vi "Feed Module (Main).vi"(7 "Name of Parent Panel":string="Main.vi", 9 "New Center Coords":T1={"Horizontal"=470, "Vertical"=200}, 10 "Config":variant, 11 "Main UI Message Queue":refnum<queue>) -> ()   [LabVIEW 2018, in "Feed Module.lvlib"]
doc: "This Continuous Measurement sample project is based on the Queued Message Handler template.\n\nThe Event Handling Loop generates messages based on user interface actions.\n\nThe Message Handling Loop processes messages generated by the Event Handling Loop, or by other messages. There are also Acquisition and Logging message handling loop subVIs, and a chart updating loop."
uses:
  Feed Module.lvlib
  support/Message Queue/Message Cluster.ctl
  <vilib>/Utility/miscctls.llb/LVPoint32TypeDef.ctl
  controls/UI Data.ctl
  controls/UI State.ctl
  Controls/Feed Module Config Cluster.ctl
  Controls/Feed Module Settings Cluster.ctl
  Ismatec ISM 831C/Controls/Ismatech Settings Cluster.ctl
  Masterflex 7550-30/Controls/Settings Cluster.ctl
  Mettler Toledo/Controls/Settings Cluster.ctl
  Bronkhorst M13 Flow Meter/Settings Cluster.ctl
  Measure Instrument/PID 2 Parameters Cluster.ctl
  Measure Instrument/PID Input Enum.ctl
  Measure Instrument/PID 2 Output Enum.ctl
  Tacmina QI/Tacmina QI DAQ Setting.ctl
  KNF Pump/Settings Cluster plus SIMDOS.ctl
  ASIA Pump/Pump Settings.ctl
  VICI M50 Party Mode/Settings Cluster.ctl
  FLOM Pump/Settings Cluster.ctl
  SSI PR Class/SSI PR Settings Cluster.ctl
  Controls/Feed Module State Cluster.ctl
  Controls/Feed Module Shared Variable Cluster.ctl
  Controls/Feed Module Display.ctl
  Sequencing/Squence Update Cluster.ctl
  support/Message Queue/Enqueue Message (Single).vi
  <vilib>/Utility/error.llb/Error Cluster From Error Code.vi
  <vilib>/ErrorRing/Error Ring.xnode
  support/User Event - Stop/User Event - Stop.lvlib
  support/Support Library.lvlib
  support/Message Queue/Message Queue.lvlib
  Measure Instrument/Feed Module Engine.lvlib
  Bronkhorst M13 Flow Meter/Bronkhorst M13 Flow Meter.lvlib
  Mettler Toledo/Mettler Toledo.lvlib
  Masterflex 7550-30/Masterflex 7550-30.lvlib
  Ismatec ISM 831C/Ismatec ISM 831C.lvlib
  Operation Window.vi
  Tacmina QI/Tacmina QI.lvlib
  KNF Pump/KNF SIMDOS.lvlib
  ASIA Pump.lvlib
  Sequencing/Sequencing Library.lvlib
  VICI M50 Party Mode/VICI M6 M50 Party Mode.lvlib
  FLOM Pump/FLOM Pump.lvlib
  support/Command Log VIs/Command Logging.lvlib
  SSI PR Class/SSI PR Pump.lvlib
panel:
  out "Pump Flow":dbl
  out "PSIG":dbl format="%#_4g"
  in  "Operation Window":bool
  out "Flow":dbl caption="g/min" format="%.2f"
  out "Ring":u16(ring)=2
  out "Log File path":path
  out "Status":string
  in  "Exit":bool
  out "kg/m^3":dbl format="%#1_4g"
  out "g":dbl format="%#_4g"
  out "C":dbl format="%#_4g"
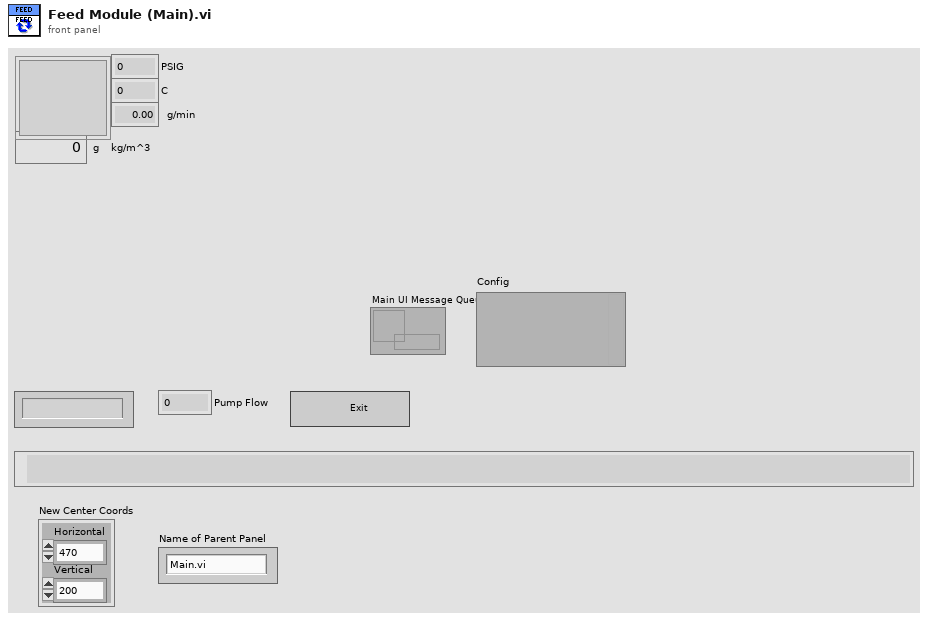
[diagram p1: front panel]
types:
  T1 = typedef "LVPoint32TypeDef.ctl" = cluster{"Horizontal":i32, "Vertical":i32}
  T2 = typedef "Feed Module.lvlib/Feed Module State Cluster.ctl" = cluster{"Shared Variables":T3, "Feed Module Config":T4}
  T3 = typedef "Feed Module.lvlib/Feed Module Shared Variable Cluster.ctl" = cluster{"PID 1 Process Variable":string, "PID 1 Output":string, "PID 1 Setpoint":string, "PID 1 Setpoint SV refnum":refnum<k21>, "PID 1 Process Variable SV refnum":refnum<k21>, "PID 1 Output SV refnum":refnum<k21>}
  T4 = typedef "Feed Module.lvlib/Feed Module Config Cluster.ctl" = cluster{"GUID":string, "Drop Coords":T1, "Process Name":string, "Settings":T5, "Settings Load Count":i32, "OP Load Count":i32}
  T5 = typedef "Feed Module.lvlib/Feed Module Settings Cluster.ctl" = cluster{"Cycle Period":dbl, "Ismatech":T6, "Masterflex":T7, "Mettler":T8, "Bronkhorst M13 Flow Meter":T9, "PID 2 Parameters":T10, "Manual Entry":dbl, "Auto?":bool, "output range":cluster{"output high":dbl, "output low":dbl}, "Bronkhorst M14":T8, "Tacmina Settings":T13, "KNF SIMDOS Settings":T14, "ASIA Pump C":T15, "VICI Settings":T16, "FLOM Settings":T17, "SSI PR Settings":T18}
  T6 = typedef "Ismatec ISM 831C.lvlib/Ismatech Settings Cluster.ctl" = cluster{"VISA resource name":refnum<visa-resource-name>, "Simulated?":bool, "Pump Number":dbl, "Reverse?":bool}
  T7 = typedef "Masterflex 7550-30.lvlib/Settings Cluster.ctl" = cluster{"VISA resource name":refnum<visa-resource-name>, "Simulated?":bool, "Pump Number":dbl, "Reverse?":bool}
  T8 = typedef "Mettler Toledo.lvlib/Settings Cluster.ctl" = cluster{"VISA resource name":refnum<visa-resource-name>, "Simulated?":bool}
  T9 = typedef "Bronkhorst M13 Flow Meter.lvlib/Settings Cluster.ctl" = cluster{"VISA resource name":refnum<visa-resource-name>, "Simulated?":bool}
  T10 = typedef "PID 2 Parameters Cluster.ctl" = cluster{"Input Device":T11, "Output Device":T12, "Setpoint":dbl, "PID gains":cluster{"proportional gain (Kc)":dbl, "integral time (Ti, min)":dbl, "derivative time (Td, min)":dbl}}
  T11 = typedef "PID Input Enum.ctl" = enum16{"Default", "Bronkhorst M13", "Bronkhorst M14", "Scale Rate of Change"}
  T12 = typedef "PID 2 Output Enum.ctl" = enum16{"Default", "Ismatec ISM 831C", "Masterflex 7550-30", "VICI", "Tacmina QI", "KNF SIMDOS", "ASIA Type C", "FLOM UI-22-11", "SSI PR"}
  T13 = typedef "Tacmina QI.lvlib/Tacmina QI DAQ Setting.ctl" = cluster{"Analog DAQ Task":refnum<k21>, "Digital DAQ Task":refnum<k21>}
  T14 = typedef "KNF SIMDOS.lvlib/Settings Cluster plus SIMDOS.ctl" = cluster{"VISA resource name":refnum<visa-resource-name>, "Simulated?":bool}
  T15 = typedef "ASIA Pump.lvlib/Pump Settings.ctl" = cluster{"ASIA Pump #":i32, "channel":i32, "Simulated":bool}
  T16 = typedef "VICI M6 M50 Party Mode.lvlib/Settings Cluster.ctl" = cluster{"VISA resource name":refnum<visa-resource-name>, "Simulated?":bool, "Pump Letter":string, "Reverse?":bool}
  T17 = typedef "FLOM Pump.lvlib/Settings Cluster.ctl" = cluster{"VISA resource name":refnum<visa-resource-name>, "Simulated?":bool, "Pump Number":dbl}
  T18 = typedef "SSI PR Pump.lvlib/SSI PR Settings Cluster.ctl" = cluster{"VISA resource name":refnum<visa-resource-name>, "Simulated?":bool}
  T19 = typedef "UI State.ctl" = enum16{"Idle", "Acquiring and Logging", "Waiting for Exit", "Waiting for Exit (Acq Stopped)", "Waiting for Exit (Log Stopped)", "Waiting for Stop", "Waiting for Stop (Acq Stopped)", "Waiting for Stop (Log Stopped)"}
  T20 = typedef "UI Data.ctl" = cluster{"Start Ref":refnum<vi>, "Trigger Ref":refnum<vi>, "Stop Ref":refnum<vi>, "Settings Ref":refnum<vi>, "Status Ref":refnum<vi>, "Exit Ref":refnum<vi>, "Data Ref":refnum<vi>}
  T21 = typedef "Feed Module.lvlib/Feed Message Queues.ctl" = cluster{"UI":refnum<queue>, "Engine":refnum<queue>, "FM Display":refnum<queue>, "OP Display":refnum<queue>}
  T22 = typedef "Feed Module.lvlib/Feed Module Display.ctl" = cluster{"Flow":dbl, "Density":dbl, "FL Temp":dbl, "Scale Value":dbl, "Pump On?":enum16{"Off", "On", "Not Initialized"}, "Cycle Period":dbl, "Input Device":T11, "Output":T12, "Pump's Pressure":dbl, "Pump's Flow ":dbl}
  T23 = cluster{"Shift":bool, "Ctrl":bool, "Alt":bool, "Cmd":bool, "Opt":bool}
  T24 = typedef "Sequencing Library.lvlib/Squence Update Cluster.ctl" = cluster{"Auto?":bool, "Manual Entry":dbl, "Setpoint":dbl}
  T25 = enum8{"Enabled", "Disabled", "Disabled and Grayed Out"}
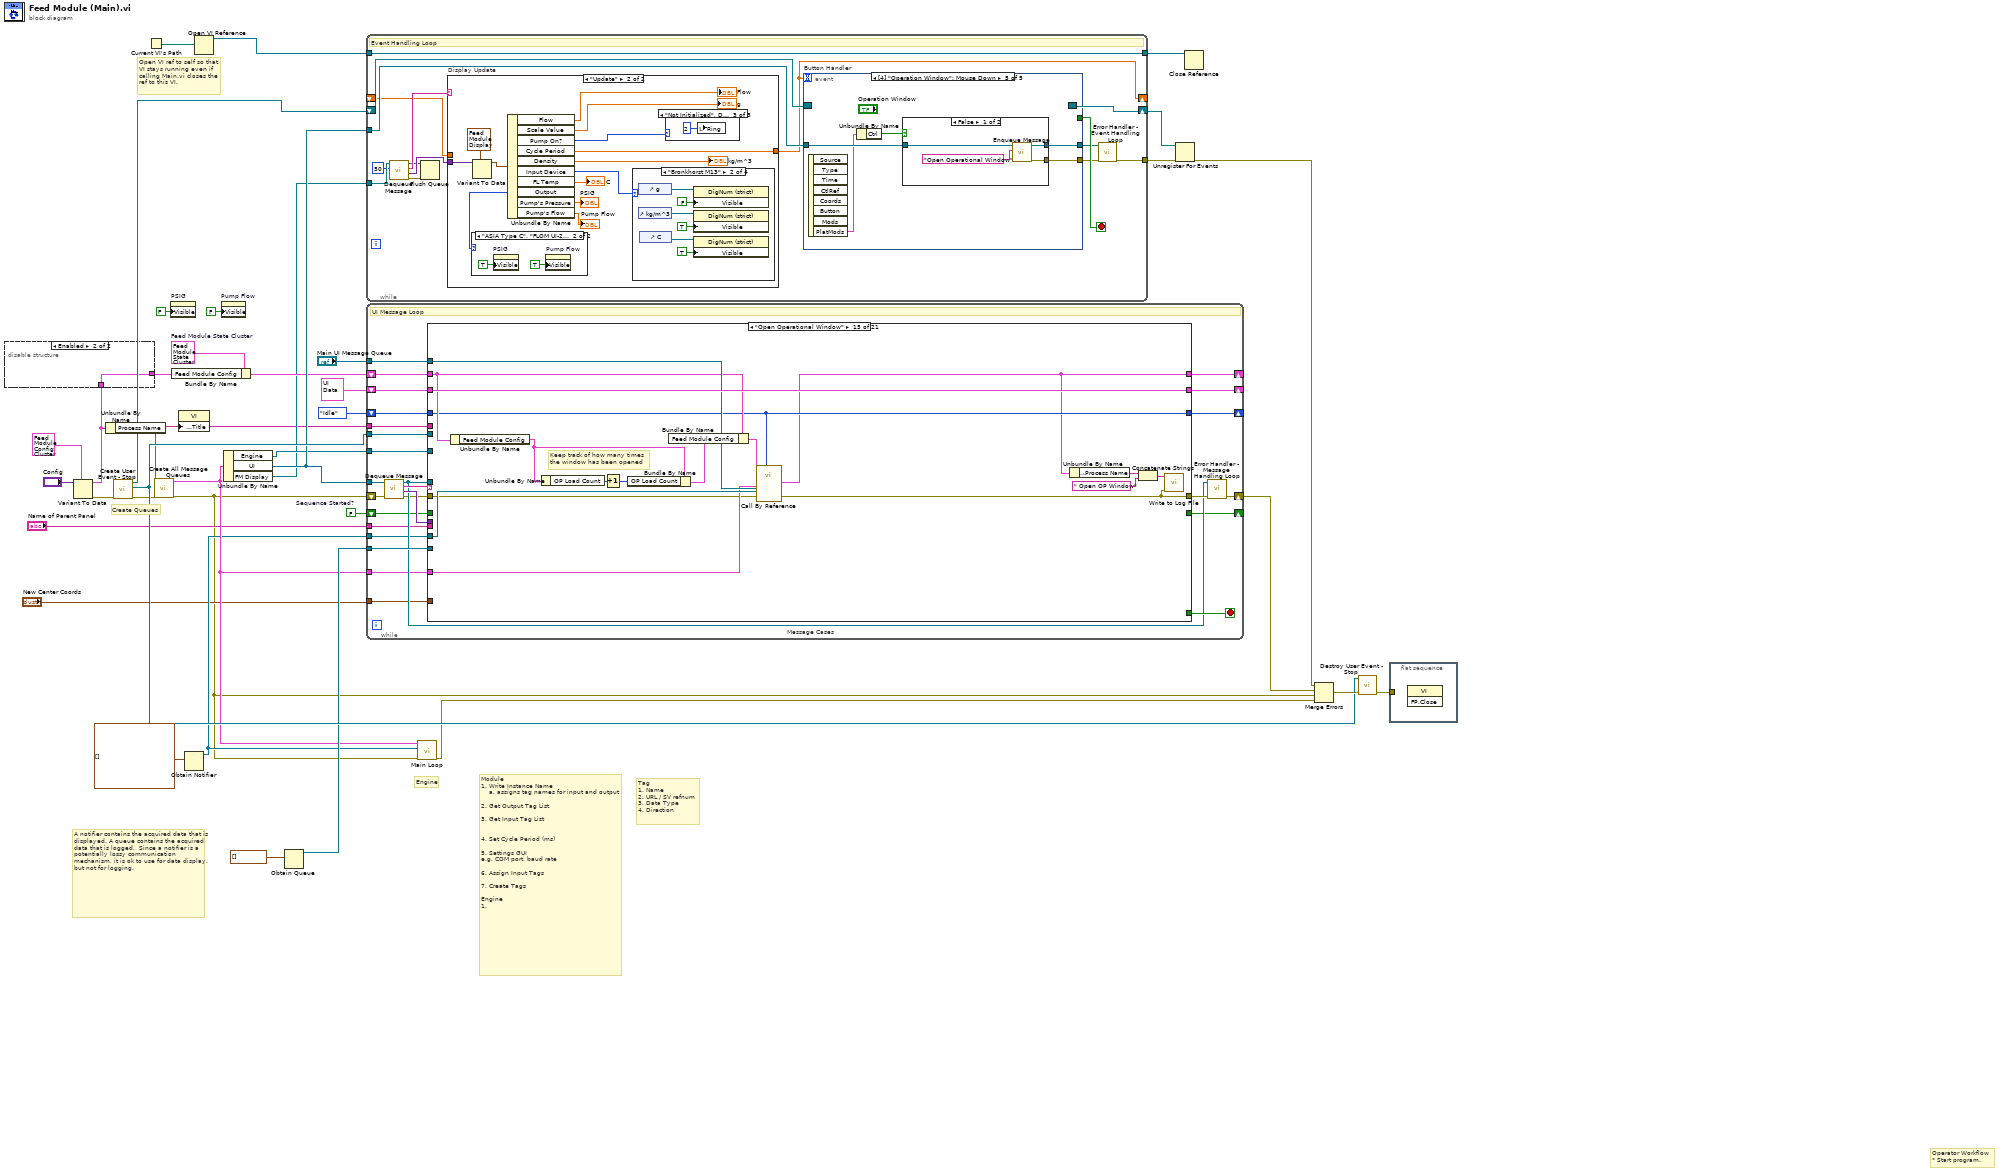
[diagram p0: block diagram]
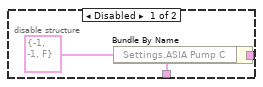
[diagram p2: hidden frame]
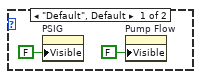
[diagram p4: hidden frame]
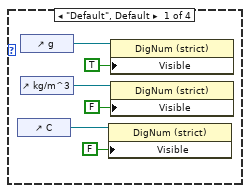
[diagram p5: hidden frame]
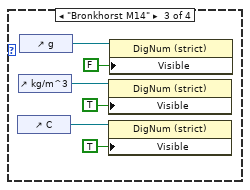
[diagram p6: hidden frame]
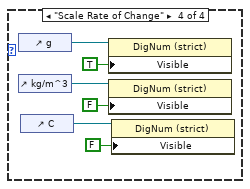
[diagram p7: hidden frame]
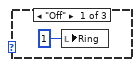
[diagram p8: hidden frame]
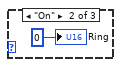
[diagram p9: hidden frame]
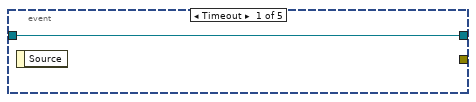
[diagram p10: hidden frame]
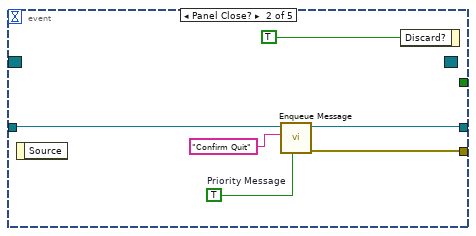
[diagram p11: hidden frame]
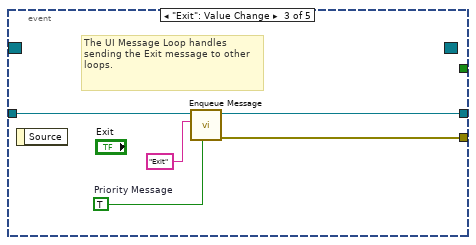
[diagram p12: hidden frame]
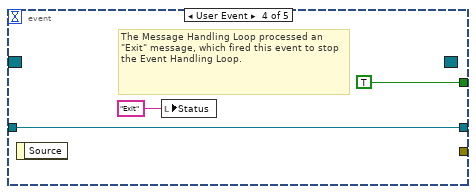
[diagram p13: hidden frame]
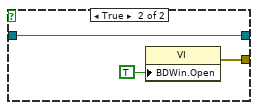
[diagram p14: hidden frame]
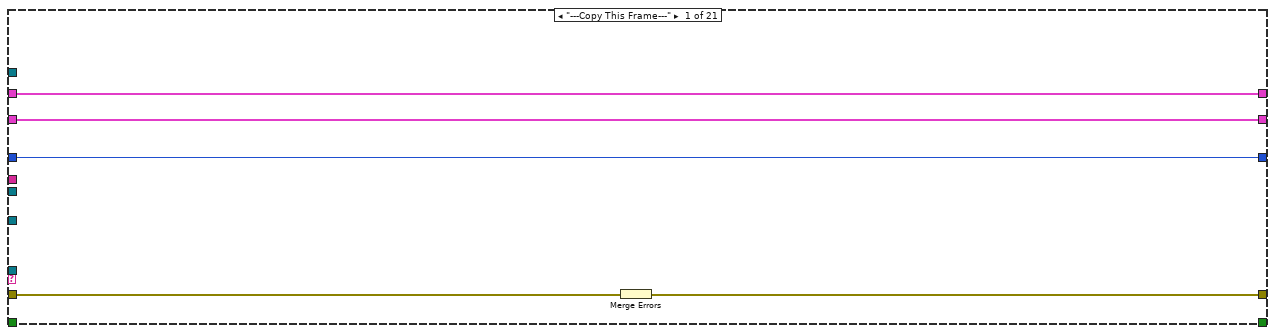
[diagram p15: hidden frame]
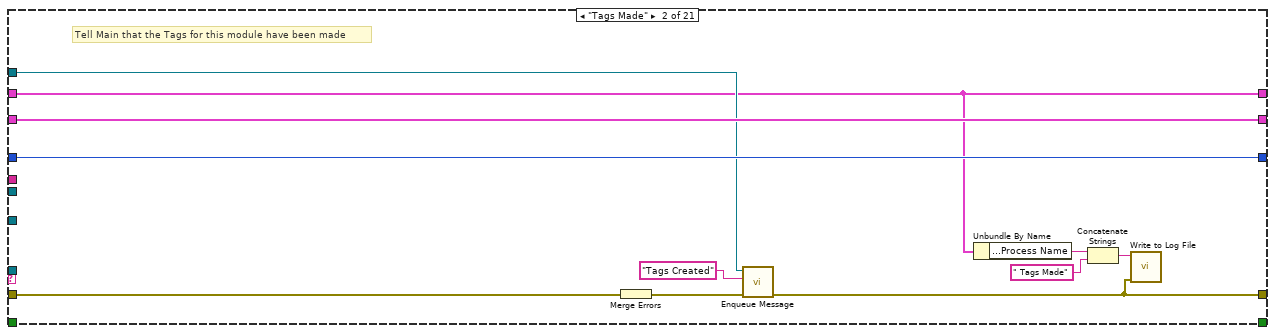
[diagram p16: hidden frame]
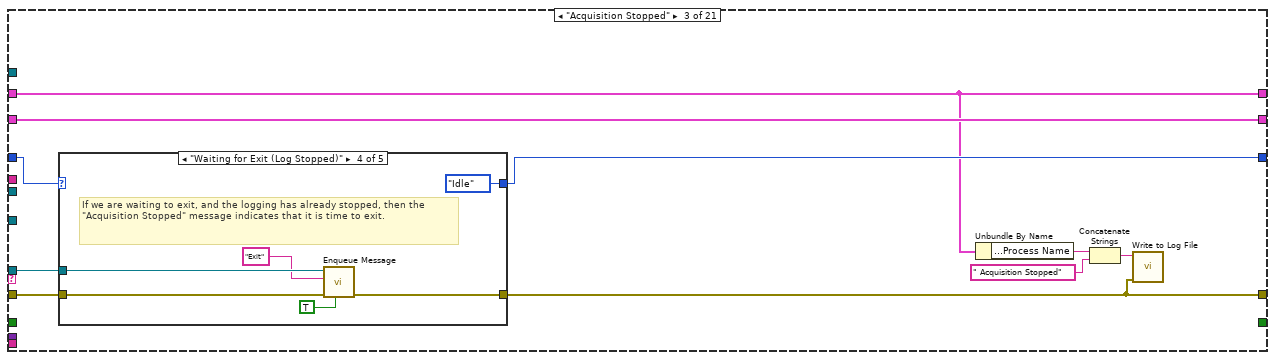
[diagram p17: hidden frame]
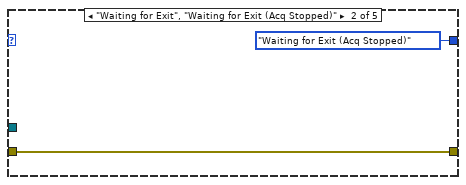
[diagram p19: hidden frame]
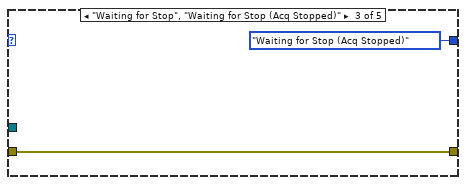
[diagram p20: hidden frame]
diagram:
  w6 = FALSE  # Sequence Started?
  w12 = T2 {"Shared Variables"={"PID 1 Process Variable"="PID1-Mettler Toledo Scale 1", "PID 1 Output"="PID1-Mettler Toledo Scale 1", "PID 1 Setpoint"="PID1-Setpoint", "PID 1 Setpoint SV refnum"="ni.var.psp://localhost/Flow Module 1/PID1-Setpoint", "PID 1 Process Variable SV refnum"="ni.var.psp://localhost/Flow Module 1/PID1-Setpoint", "PID 1 Output SV refnum"="ni.var.psp://localhost/Flow Module 1/PID1-Setpoint"}, "Feed Module Config"={"GUID"="", "Drop Coords"={"Horizontal"=0, "Vertical"=0}, "Process Name"="", "Settings"={"Cycle Period"=500.0, "Ismatech"={"VISA resource name"="", "Simulated?"=TRUE, "Pump Number"=1.0, "Reverse?"=FALSE}, "Masterflex"={"VISA resource name"="", "Simulated?"=TRUE, "Pump Number"=1.0, "Reverse?"=FALSE}, "Mettler"={"VISA resource name"="", "Simulated?"=FALSE}, "Bronkhorst M13 Flow Meter"={"VISA resource name"="", "Simulated?"=TRUE}, "PID 2 Parameters"={"Input Device"=enum."Default", "Output Device"=enum."Default", "Setpoint"=0.0, "PID gains"={"proportional gain (Kc)"=1.0, "integral time (Ti, min)"=0.01, "derivative time (Td, min)"=0.0}}, "Manual Entry"=0.0, "Auto?"=TRUE, "output range"={"output high"=100.0, "output low"=0.0}, "Bronkhorst M14"={"VISA resource name"="", "Simulated?"=FALSE}, "Tacmina Settings"={"Analog DAQ Task"="", "Digital DAQ Task"=""}, "KNF SIMDOS Settings"={"VISA resource name"="", "Simulated?"=TRUE}, "ASIA Pump C"={"ASIA Pump #"=0, "channel"=0, "Simulated"=FALSE}, "VICI Settings"={"VISA resource name"="", "Simulated?"=TRUE, "Pump Letter"="", "Reverse?"=FALSE}, "FLOM Settings"={"VISA resource name"="", "Simulated?"=TRUE, "Pump Number"=0.0}, "SSI PR Settings"={"VISA resource name"="", "Simulated?"=FALSE}}, "Settings Load Count"=0, "OP Load Count"=0}}  # Feed Module State Cluster
  # "Create Queues"
  # "Open VI ref to self so that\nVI stays running even if\ncalling Main.vi closes the\nref to this VI."
  # "Engine"
  # "Operator Workflow\n* Start program."
  # "Module \n1. Write Instance Name\n    a. assigns tag names for input and output\n\n2. Get Output Tag List\n\n3. Get Input Tag List\n\n\n4. Set Cycle Period (ms)\n\n5. Settings GUI\ne.g. COM port, baud rate\n\n6. Assign Input Tags\n\n7. Create Tags\n\nEngine\n1."
  # "Tag\n1. Name\n2. URL / SV refnum\n3. Data Type\n4. Direction"
  # "A notifier contains the acquired data that is displayed. A queue contains the acquired data that is logged.  Since a notifier is a potentially lossy communication mechanism, it is ok to use for data display, but not for logging."
  n1 = Variant To Data(type=T4 {"GUID"="", "Drop Coords"={"Horizontal"=0, "Vertical"=0}, "Process Name"="", "Settings"={"Cycle Period"=500.0, "Ismatech"={"VISA resource name"="", "Simulated?"=TRUE, "Pump Number"=1.0, "Reverse?"=FALSE}, "Masterflex"={"VISA resource name"="", "Simulated?"=TRUE, "Pump Number"=1.0, "Reverse?"=FALSE}, "Mettler"={"VISA resource name"="", "Simulated?"=FALSE}, "Bronkhorst M13 Flow Meter"={"VISA resource name"="", "Simulated?"=TRUE}, "PID 2 Parameters"={"Input Device"=enum."Default", "Output Device"=enum."Default", "Setpoint"=0.0, "PID gains"={"proportional gain (Kc)"=1.0, "integral time (Ti, min)"=0.01, "derivative time (Td, min)"=0.0}}, "Manual Entry"=0.0, "Auto?"=TRUE, "output range"={"output high"=100.0, "output low"=0.0}, "Bronkhorst M14"={"VISA resource name"="", "Simulated?"=FALSE}, "Tacmina Settings"={"Analog DAQ Task"="", "Digital DAQ Task"=""}, "KNF SIMDOS Settings"={"VISA resource name"="", "Simulated?"=TRUE}, "ASIA Pump C"={"ASIA Pump #"=0, "channel"=0, "Simulated"=FALSE}, "VICI Settings"={"VISA resource name"="", "Simulated?"=TRUE, "Pump Letter"="", "Reverse?"=FALSE}, "FLOM Settings"={"VISA resource name"="", "Simulated?"=TRUE, "Pump Number"=0.0}, "SSI PR Settings"={"VISA resource name"="", "Simulated?"=FALSE}}, "Settings Load Count"=0, "OP Load Count"=0} ("Feed Module Config"), Variant="Config") -> (data=w2:T4, error out=w15:errorcluster)  [unwired: 1 in]
  n2 = disable-structure shown="Enabled" {
    disable-tunnel: w2 -> [w40 w42]
    disable-tunnel: [w39 w42] -> w1
    frame Disabled {
      n3 = Bundle By Name(cluster=w40, "Settings.ASIA Pump C"=T15 {"ASIA Pump #"=-1, "channel"=-1, "Simulated"=FALSE}) -> (w39:T4)
    }
    frame Enabled {
    }
  }
  n4 = Unbundle By Name(w2) -> ("Process Name"=w9:string)
  n5 = call "Create User Event - Stop.vi"("error in (no error)"=w15) -> ("error out"=w33:errorcluster, "User Event - Stop"=w34:refnum<user-event>, "Stop Event Registration Refnum"=w35:refnum<event-registration>)  [unwired: 8 in]
  n6 = Current VI's Path() -> (path=w18:path)
  n7 = call "Create All Message Queues.vi"("error in (no error)"=w33, "Process Name"=w9) -> ("error out"=w5:errorcluster, "Message Queues"=w22:T21)  [unwired: 8 in]
  n8 = property on="PSIG" class="DigNum (strict)"("Visible"=FALSE) -> ()  [unwired: 2 in, 2 out]
  n9 = Bundle By Name(cluster=w12, "Feed Module Config"=w1) -> (w16:T2)
  n10 = property class="VI"("Front Panel.Title"=w9) -> ()  [unwired: 2 in, 2 out]
  n11 = Obtain Notifier(notification data type=waveform(dbl)[] []) -> (notifier out=w21:refnum<notifier>)  [unwired: 3 in, 2 out]
  n12 = Open VI Reference(vi path=w18) -> (vi reference=w19:refnum<vi>)  [unwired: 5 in, 1 out]
  n13 = property on="Pump Flow" class="DigNum (strict)"("Visible"=FALSE) -> ()  [unwired: 2 in, 2 out]
  n14 = Unbundle By Name(w22) -> ("Engine"=w25:refnum<queue>, "UI"=w29:refnum<queue>, "FM Display"=w11:refnum<queue>)
  n15 = Obtain Queue(element data type=waveform(dbl)[] []) -> (queue out=w24:refnum<queue>)  [unwired: 4 in, 2 out]
  n16 = while {
    tunnel: w29 -> [w52]
    tunnel: [w54] -> w37
    shift-right: [w53] -> w31
    shift-left: w35 -> [w58]
    tunnel: [w51] -> w20
    tunnel: w19 -> [w51]
    tunnel: w11 -> [w50]
    shift-right: [w47] -> _
    shift-left: _ -> [w46]
    stop <- w57 stop-if-true
    # "Event Handling Loop"
    n17 = call "Dequeue Message.vi"("timeout in ms (-1)"=50, "Message Queue"=w50) -> ("error out"=w43:errorcluster, "Message Data"=w48:variant, "Message"=w49:string, "dup Message Queue"=w44:refnum<queue>)  [unwired: 6 in]
    n18 = Flush Queue(queue=w44, error in (no error)=w43) -> ()  [unwired: 3 out]
    n19 = case "Display Update" shown="\"Update\"" w49 {
      tunnel: w48 -> [_ w72]
      tunnel: [w59 w66] -> w47
      tunnel: w46 -> [w59 _]
      frame "False", Default {
      }
      frame "Update" {
        n20 = Variant To Data(type=T22 {"Flow"=0.0, "Density"=0.0, "FL Temp"=0.0, "Scale Value"=0.0, "Pump On?"=enum."Off", "Cycle Period"=500.0, "Input Device"=enum."Bronkhorst M13", "Output"=enum."Default", "Pump's Pressure"=0.0, "Pump's Flow "=0.0}, Variant=w72) -> (data=w70:T22)  [unwired: 1 in, 1 out]
        n21 = Unbundle By Name(w70) -> ("Flow"=→"Flow":dbl, "Scale Value"=→"g":dbl, "Pump On?"=w67:enum16{"Off", "On", "Not Initialized"}, "Cycle Period"=w66:dbl, "Density"=→"kg/m^3":dbl, "Input Device"=w65:T11, "FL Temp"=→"C":dbl, "Output"=w62:T12, "Pump's Pressure"=→"PSIG":dbl, "Pump's Flow"=→"Pump Flow":dbl)
        n22 = case shown="\"ASIA Type C\", \"FLOM UI-22-11\"" w62 {
          frame "Default", Default {
            n23 = property on="PSIG" class="DigNum (strict)"("Visible"=FALSE) -> ()  [unwired: 2 in, 2 out]
            n24 = property on="Pump Flow" class="DigNum (strict)"("Visible"=FALSE) -> ()  [unwired: 2 in, 2 out]
          }
          frame "ASIA Type C", "FLOM UI-22-11" {
            n25 = property on="PSIG" class="DigNum (strict)"("Visible"=TRUE) -> ()  [unwired: 2 in, 2 out]
            n26 = property on="Pump Flow" class="DigNum (strict)"("Visible"=TRUE) -> ()  [unwired: 2 in, 2 out]
          }
        }
        n27 = case shown="\"Bronkhorst M13\"" w65 {
          frame "Default", Default {
            n28 = control-ref of="C"() -> (w78:refnum<vi>)
            n29 = control-ref of="g"() -> (w81:refnum<vi>)
            n30 = control-ref of="kg/m^3"() -> (w82:refnum<vi>)
            n31 = property class="DigNum (strict)"(reference=w78, "Visible"=FALSE) -> ()  [unwired: 1 in, 2 out]
            n32 = property class="DigNum (strict)"(reference=w81, "Visible"=TRUE) -> ()  [unwired: 1 in, 2 out]
            n33 = property class="DigNum (strict)"(reference=w82, "Visible"=FALSE) -> ()  [unwired: 1 in, 2 out]
          }
          frame "Bronkhorst M13" {
            n34 = control-ref of="g"() -> (w87:refnum<vi>)
            n35 = control-ref of="kg/m^3"() -> (w88:refnum<vi>)
            n36 = control-ref of="C"() -> (w84:refnum<vi>)
            n37 = property class="DigNum (strict)"(reference=w87, "Visible"=FALSE) -> ()  [unwired: 1 in, 2 out]
            n38 = property class="DigNum (strict)"(reference=w88, "Visible"=TRUE) -> ()  [unwired: 1 in, 2 out]
            n39 = property class="DigNum (strict)"(reference=w84, "Visible"=TRUE) -> ()  [unwired: 1 in, 2 out]
          }
          frame "Bronkhorst M14" {
            n40 = control-ref of="C"() -> (w89:refnum<vi>)
            n41 = control-ref of="kg/m^3"() -> (w94:refnum<vi>)
            n42 = control-ref of="g"() -> (w93:refnum<vi>)
            n43 = property class="DigNum (strict)"(reference=w94, "Visible"=TRUE) -> ()  [unwired: 1 in, 2 out]
            n44 = property class="DigNum (strict)"(reference=w89, "Visible"=TRUE) -> ()  [unwired: 1 in, 2 out]
            n45 = property class="DigNum (strict)"(reference=w93, "Visible"=FALSE) -> ()  [unwired: 1 in, 2 out]
          }
          frame "Scale Rate of Change" {
            n46 = control-ref of="g"() -> (w99:refnum<vi>)
            n47 = control-ref of="kg/m^3"() -> (w100:refnum<vi>)
            n48 = control-ref of="C"() -> (w95:refnum<vi>)
            n49 = property class="DigNum (strict)"(reference=w99, "Visible"=TRUE) -> ()  [unwired: 1 in, 2 out]
            n50 = property class="DigNum (strict)"(reference=w100, "Visible"=FALSE) -> ()  [unwired: 1 in, 2 out]
            n51 = property class="DigNum (strict)"(reference=w95, "Visible"=FALSE) -> ()  [unwired: 1 in, 2 out]
          }
        }
        n52 = case shown="\"Not Initialized\", Default" w67 {
          frame "Off" {
            n53 = local write "Ring"(u16 1 ("Ring")) -> ()
          }
          frame "On" {
            "Ring" <- u16 0 ("Ring")
          }
          frame "Not Initialized", Default {
            n54 = local write "Ring"(u16 2 ("Ring")) -> ()
          }
        }
      }
    }
    n55 = event "Button Handler" shown="[4] \"Operation Window\": Mouse Down" {
      selector: w58 -> [_ _ _ _ _]
      dyn-events: [_ _ _ _ _] -> w53
      timeout: w47 -> [_ _ _ _ _]
      tunnel: [_ _ _ TRUE ("Discard?") _] -> w57
      tunnel: w52 -> [w104 w107 w112 w116 w121]
      tunnel: [_ w105 w115 _ w123] -> w55
      tunnel: [w104 w106 w111 w116 w122] -> w56
      event Timeout {
        n56 = event-data() -> ()  [unwired: 1 in, 1 out]
      }
      event Panel Close? {
        w108 = TRUE  # Priority Message
        n57 = event-data() -> ()  [unwired: 1 in, 1 out]
        n58 = call-poly "Enqueue Message.vi"("Priority Message? (F)"=w108, "Message"="Confirm Quit", "Message Queue"=w107) -> ("error out"=w105:errorcluster, "dup Message Queue"=w106:refnum<queue>)  [unwired: 7 in]
        n59 = event-data("Discard?"=TRUE) -> ()  [unwired: 1 in, 1 out]
      }
      event "Exit": Value Change {
        w113 = TRUE  # Priority Message
        # "The UI Message Loop handles sending the Exit message to other loops."
        n60 = event-data() -> ()  [unwired: 1 in, 1 out]
        n61 = call-poly "Enqueue Message.vi"("Priority Message? (F)"=w113, "Message"="Exit", "Message Queue"=w112) -> ("error out"=w115:errorcluster, "dup Message Queue"=w111:refnum<queue>)  [unwired: 7 in]
      }
      event User Event {
        # "The Message Handling Loop processed an \"Exit\" message, which fired this event to stop the Event Handling Loop."
        n62 = event-data() -> ()  [unwired: 1 in, 1 out]
        n63 = local write "Status"("Exit" ("Exit String")) -> ()
      }
      event "Operation Window": Mouse Down {
        n64 = event-data() -> ("PlatMods"=w120:T23)  [unwired: 1 in, 7 out]
        n65 = Unbundle By Name(w120) -> ("Ctrl"=w119:bool)
        n66 = case shown="False" w119 {
          tunnel: [w127 w128] -> w123
          tunnel: [w126 w129] -> w122
          tunnel: w121 -> [w125 w129]
          frame False {
            n67 = call-poly "Enqueue Message.vi"("Message"="Open Operational Window", "Message Queue"=w125) -> ("error out"=w127:errorcluster, "dup Message Queue"=w126:refnum<queue>)  [unwired: 8 in]
          }
          frame True {
            n68 = property class="VI"("BDWin.Open"=TRUE ("Block Diagram Window:Open")) -> (error out=w128:errorcluster)  [unwired: 2 in, 1 out]
          }
        }
      }
    }
    n69 = call "Error Handler - Event Handling Loop.vi"("error in (no error)"=w55, "Message Queue"=w56) -> ("dup error in"=w54:errorcluster)  [unwired: 8 in, 1 out]
  }
  n70 = while {
    tunnel: w29 -> [w151]
    tunnel: w34 -> [w155]
    shift-right: [w145] -> w38
    shift-left: w5 -> [w154]
    shift-right: [w150] -> _
    shift-left: w16 -> [w133]
    shift-right: [w148] -> _
    shift-left: T20 {"Start Ref"=refnum, "Trigger Ref"=refnum, "Stop Ref"=refnum, "Settings Ref"=refnum, "Status Ref"=refnum, "Exit Ref"=refnum, "Data Ref"=refnum} ("Measurement UI Controls") -> [w149]
    tunnel: w21 -> [w135]
    tunnel: w24 -> [w147]
    shift-right: [w143] -> _
    shift-left: UI_State."Idle" ("UI State") -> [w137]
    tunnel: w25 -> [w142]
    tunnel: w22 -> [w134]
    tunnel: "Main UI Message Queue" -> [w138]
    tunnel: "Name of Parent Panel" -> [w141]
    tunnel: w9 -> [w140]
    tunnel: "New Center Coords" -> [w139]
    shift-right: [w131] -> _
    shift-left: w6 -> [w132]
    stop <- w156 stop-if-true
    # "UI Message Loop"
    n71 = call "Dequeue Message.vi"("error in (no error)"=w154, "Message Queue"=w151) -> ("error out"=w136:errorcluster, "Message Data"=w152:variant, "Message"=w153:string, "dup Message Queue"=w144:refnum<queue>)  [unwired: 6 in]
    n72 = case "Message Cases" shown="\"Open Operational Window\"" w153 {
      selector: w153 -> [_ _ _ _ _ _ _ _ _ _ _ _ _ _ _ _ _ _ _ _ w582]
      tunnel: w144 -> [_ _ w178 _ w242 _ w298 w314 w345 w370 _ w408 w429 w439 _ w488 _ _ w559 _ _]
      tunnel: w136 -> [w161 w172 w179 w213 w241 w267 w283 w313 w349 w374 w393 w403 _ w440 w467 w486 w507 w524 w544 w576 _]
      tunnel: [w160 w163 w174 w204 w236 w268 w275 w302 w334 w352 w393 w395 w416 w435 w463 w480 w505 w519 w536 w563 w584] -> w146
      tunnel: [_ _ _ _ _ _ _ _ _ TRUE _ _ _ _ _ _ _ _ _ _ _] -> w156
      tunnel: w152 -> [_ _ _ _ _ w270 _ _ w348 w358 _ _ w427 _ _ _ _ _ _ w575 _]
      tunnel: w155 -> [_ _ _ _ _ _ _ _ _ w373 _ _ _ _ _ _ _ _ _ _ _]
      tunnel: [w159 w162 w173 w203 w235 w273 w274 w301 w336 w351 w392 w394 w415 w434 w462 w479 w504 w518 w535 w562 w583] -> w150
      tunnel: w149 -> [w158 w171 w182 w218 w244 w272 w295 w311 w350 w371 w391 w404 w433 w443 w478 w503 w512 w529 w556 w572 w589]
      tunnel: [w158 w171 w182 w218 w244 w272 w295 w311 w350 w371 w390 w404 w433 w443 w478 w503 w512 w529 w556 w572 w589] -> w148
      tunnel: w147 -> [_ _ _ _ _ _ _ _ _ w365 _ _ _ _ _ _ _ _ _ _ _]
      tunnel: w137 -> [w157 w170 w181 w217 w243 w266 w284 _ w340 _ _ _ w432 w442 w468 _ _ _ w545 w567 w588]
      tunnel: [w157 w170 w180 w217 w240 w266 w285 UI_State."Acquiring and Logging" ("UI State") w340 UI_State."Idle" ("UI State") UI_State."Idle" ("UI State") UI_State."Idle" ("UI State") w432 w441 w468 UI_State."Acquiring and Logging" ("UI State") UI_State."Acquiring and Logging" ("UI State") UI_State."Acquiring and Logging" ("UI State") w546 w567 w588] -> w143
      tunnel: w142 -> [_ _ _ w212 _ _ w282 _ _ w363 _ _ _ _ _ _ w510 w527 w543 _ _]
      tunnel: w141 -> [_ _ _ _ _ _ _ _ _ _ _ w402 _ _ _ _ _ _ _ _ _]
      tunnel: w140 -> [_ _ _ _ _ _ _ _ _ _ _ w399 _ _ _ _ _ _ _ _ _]
      tunnel: w139 -> [_ _ _ _ _ _ _ _ _ _ _ w401 _ _ _ _ _ _ _ _ _]
      tunnel: w138 -> [_ w168 _ _ _ _ _ _ _ w356 _ _ _ _ w477 _ _ _ _ _ _]
      tunnel: w135 -> [_ _ _ _ _ _ _ _ _ w369 _ _ _ _ w476 _ _ _ _ _ _]
      tunnel: w134 -> [_ _ _ w216 _ _ _ _ _ _ _ _ _ _ w475 _ _ _ _ _ _]
      tunnel: w133 -> [w159 w162 w173 w203 w235 w273 w274 w301 w336 w351 w392 w394 w431 w434 w471 w479 w504 w518 w535 w562 w583]
      tunnel: w132 -> [_ _ _ _ _ _ _ w310 _ _ _ _ _ _ _ _ _ _ _ _ _]
      tunnel: [_ _ _ _ _ _ _ w307 _ _ _ _ _ _ _ _ _ _ _ _ _] -> w131
      frame "---Copy This Frame---" {
        # "Duplicate this frame when creating new messages.  Change this comment in the duplicated frame to describe this message."
        n73 = Merge Errors(w161) -> (w160:errorcluster)
      }
      frame "Tags Made" {
        # "Tell Main that the Tags for this module have been made"
        # "Duplicate this frame when creating new messages.  Change this comment in the duplicated frame to describe this message."
        n74 = Merge Errors(w172) -> (w167:errorcluster)
        n75 = call-poly "Enqueue Message.vi"("error in (no error)"=w167, "Message"="Tags Created", "Message Queue"=w168) -> ("error out"=w163:errorcluster)  [unwired: 7 in, 1 out]
        n76 = Unbundle By Name(w162) -> ("Feed Module Config.Process Name"=w166:string)
        n77 = Concatenate Strings(w166, " Tags Made" ("text")) -> (w164:string)
        n78 = call "Write to Log File.vi"("error in"=w163, "text"=w164) -> ()  [unwired: 9 in, 1 out]
      }
      frame "Acquisition Stopped" {
        # "Logic for determining what action to take when the acquisition has stopped."
        n79 = case shown="\"Waiting for Exit (Log Stopped)\"" w181 {
          selector: w181 -> [w184 _ _ _ _]
          tunnel: [w184 UI_State."Waiting for Exit (Acq Stopped)" ("UI State") UI_State."Waiting for Stop (Acq Stopped)" ("UI State") UI_State."Idle" ("UI State") UI_State."Idle" ("UI State")] -> w180
          tunnel: w179 -> [w183 w185 w187 w193 w199]
          tunnel: [w183 w185 w187 w192 w198] -> w174
          tunnel: w178 -> [_ _ _ w191 w197]
          frame Default {
          }
          frame "Waiting for Exit", "Waiting for Exit (Acq Stopped)" {
          }
          frame "Waiting for Stop", "Waiting for Stop (Acq Stopped)" {
          }
          frame "Waiting for Exit (Log Stopped)" {
            # "If we are waiting to exit, and the logging has already stopped, then the \"Acquisition Stopped\" message indicates that it is time to exit."
            n80 = call-poly "Enqueue Message.vi"("Priority Message? (F)"=TRUE, "error in (no error)"=w193, "Message"="Exit", "Message Queue"=w191) -> ("error out"=w192:errorcluster)  [unwired: 6 in, 1 out]
          }
          frame "Waiting for Stop (Log Stopped)" {
            # "If we are waiting to stop, and the logging has already stopped, then the \"Acquisition Stopped\" message indicates that it is time to stop."
            n81 = call-poly "Enqueue Message.vi"("error in (no error)"=w199, "Message Data"="Ready..." ("Message"), "Message"="Update Status", "Message Queue"=w197) -> ("error out"=w198:errorcluster)  [unwired: 6 in, 1 out]
          }
        }
        n82 = Unbundle By Name(w173) -> ("Feed Module Config.Process Name"=w177:string)
        n83 = Concatenate Strings(w177, " Acquisition Stopped" ("text")) -> (w175:string)
        n84 = call "Write to Log File.vi"("error in"=w174, "text"=w175) -> ()  [unwired: 9 in, 1 out]
      }
      frame "Broadcast Settings" {
        # "If this is the first time the settings\nhave been sent and the setpoint is 0 \nmove the engine into the pause state"
        # "Send the settings to the engine"
        # "Send the 'Update Settings' message to the Logging and Acquisition message loops."
        n85 = Unbundle By Name(w203) -> ("Feed Module Config.Settings.Cycle Period"=w214:dbl)
        n86 = call "Cycle Period FGV.vi"("Write"=TRUE, "Cycle Period In (ms)"=w214) -> ()  [unwired: 8 in, 2 out]
        n87 = Unbundle By Name(w203) -> ("Feed Module Config.Settings.Auto?"=w208:bool)
        n88 = case shown="True" w208 {
          tunnel: [w219 w224] -> w210
          tunnel: [w220 w223] -> w209
          tunnel: w203 -> [w221 w222]
          frame False {
            n89 = Unbundle By Name(w221) -> ("Feed Module Config.Settings.Manual Entry"=w220:dbl, "Feed Module Config.Settings.PID 2 Parameters.Input Device"=w219:T11)
          }
          frame True {
            n90 = Unbundle By Name(w222) -> ("Feed Module Config.Settings.PID 2 Parameters.Setpoint"=w223:dbl, "Feed Module Config.Settings.PID 2 Parameters.Input Device"=w224:T11)
          }
        }
        n91 = call "Broadcast Settings.vi"("error in (no error)"=w213, "Message Queues"=w216, "Feed Module State Cluster in"=w203) -> ("error out"=w211:errorcluster)  [unwired: 8 in]
        n92 = case shown="\"Bronkhorst M13\"..\"Scale Rate of Change\"" w210 {
          tunnel: w211 -> [w225 w229]
          tunnel: w212 -> [_ w228]
          tunnel: [w225 w227] -> w204
          tunnel: w209 -> [_ w226]
          frame "Default", Default {
          }
          frame "Bronkhorst M13".."Scale Rate of Change" {
            n93 = case shown="0" w226 {
              tunnel: w229 -> [w230 w234]
              tunnel: w228 -> [_ w233]
              tunnel: [w230 w232] -> w227
              frame Default {
              }
              frame 0 {
                n94 = call-poly "Enqueue Message.vi"("error in (no error)"=w234, "Message"="Pause", "Message Queue"=w233) -> ("error out"=w232:errorcluster)  [unwired: 7 in, 1 out]
              }
            }
          }
        }
        n95 = Unbundle By Name(w203) -> ("Feed Module Config.Settings"=w202:T5)
        n96 = Unbundle By Name(w203) -> ("Feed Module Config.Process Name"=w207:string)
        n97 = Flatten To XML(anything=w202) -> (xml string=w201:string)
        n98 = Concatenate Strings(w207, " Broadcast Settings" ("text"), w201) -> (w205:string)
        n99 = call "Write to Log File.vi"("error in"=w204, "text"=w205) -> ()  [unwired: 9 in, 1 out]
      }
      frame "Confirm Quit" {
        # "Confirm Quit - Message that can confirm whether or not the user wants to exit the application."
        n100 = case shown="\"Acquiring and Logging\"" w243 {
          tunnel: w242 -> [w249 w255]
          tunnel: w241 -> [w248 w253]
          tunnel: [w245 w252] -> w236
          tunnel: [UI_State."Idle" ("UI State") w251] -> w240
          frame Default {
            # "If 'Confirm Quit' comes in while the system is idle, there is no need for a confirmation message."
            n101 = call-poly "Enqueue Message.vi"("Priority Message? (F)"=TRUE, "error in (no error)"=w248, "Message"="Exit", "Message Queue"=w249) -> ("error out"=w245:errorcluster)  [unwired: 6 in, 1 out]
          }
          frame "Acquiring and Logging" {
            n102 = Two Button Dialog(message="Are you sure you want to quit while the acquisition is running?" ("Confirm Quit Message"), 1:"No" ("No"), 2:"Yes" ("Yes")) -> (T button?=w254:bool)
            n103 = case shown="True" w254 {
              tunnel: w255 -> [_ w265]
              tunnel: w253 -> [w259 w264]
              tunnel: [w259 w263] -> w252
              tunnel: [UI_State."Acquiring and Logging" ("UI State") UI_State."Waiting for Exit" ("UI State")] -> w251
              frame False {
                # "User did not want to quit."
              }
              frame True {
                n104 = call-poly "Enqueue Message.vi"("error in (no error)"=w264, "Message"="Stop", "Message Queue"=w265) -> ("error out"=w263:errorcluster)  [unwired: 7 in, 1 out]
              }
            }
          }
        }
        n105 = Unbundle By Name(w235) -> ("Feed Module Config.Process Name"=w239:string)
        n106 = Concatenate Strings(w239, " Quit" ("text")) -> (w237:string)
        n107 = call "Write to Log File.vi"("error in"=w236, "text"=w237) -> ()  [unwired: 9 in, 1 out]
      }
      frame "Display Log File Path" {
        n108 = Variant To Data(error in=w267, type=path "", Variant=w270) -> (data=→"Log File path":path, error out=w268:errorcluster)
      }
      frame "E-Stop" {
        # "E-Stop pauses the engine"
        # "Message Acquisition and Logging loops to stop"
        # "Enable: Start, Exit, Settings\nDisable: Stop"
        # "Stop the pumps."
        n109 = Unbundle By Name(w295) -> ("Trigger Ref"=w286:refnum<vi>, "Stop Ref"=w287:refnum<vi>, "Start Ref"=w290:refnum<vi>, "Exit Ref"=w289:refnum<vi>, "Settings Ref"=w288:refnum<vi>)
        n110 = call-poly "Enqueue Message.vi"("error in (no error)"=w283, "Message Data"="Ready..." ("Ready..."), "Message"="Update Status", "Message Queue"=w298) -> ("error out"=w280:errorcluster)  [unwired: 6 in, 1 out]
        n111 = Build Array(w290, w289, w288) -> (w293:refnum<vi>[])
        n112 = Build Array(w286, w287) -> (w292:refnum<vi>[])
        n113 = call-poly "Enqueue Message.vi"("error in (no error)"=w280, "Message"="Pause", "Message Queue"=w282) -> ("error out"=w279:errorcluster)  [unwired: 7 in, 1 out]
        n114 = call "Set Enable State on Multiple Controls.vi"("Enable?"=FALSE, "Controls"=w292) -> ()  [unwired: 10 in]
        n115 = call "Set Enable State on Multiple Controls.vi"("Enable?"=TRUE, "Controls"=w293) -> ()  [unwired: 10 in]
        n116 = case shown="\"Waiting for Exit\"" w284 {
          selector: w284 -> [_ w300]
          tunnel: [UI_State."Waiting for Stop" ("UI State") w300] -> w285
          frame Default {
          }
          frame "Waiting for Exit" {
          }
        }
        n117 = Merge Errors(w279) -> (w275:errorcluster)
        n118 = Unbundle By Name(w274) -> ("Feed Module Config.Process Name"=w278:string)
        n119 = Concatenate Strings(w278, " E-STOP" ("text")) -> (w276:string)
        n120 = call "Write to Log File.vi"("error in"=w275, "text"=w276) -> ()  [unwired: 9 in, 1 out]
      }
      frame "Sequence Start" {
        # "Clear chart"
        # "Message Acquisition and Logging loops to start"
        # "Enable: Stop\nDisable: Start, Exit, Settings"
        # "Stop the pumps."
        n121 = Unbundle By Name(w311) -> ("Trigger Ref"=w318:refnum<vi>, "Stop Ref"=w319:refnum<vi>, "Start Ref"=w322:refnum<vi>, "Exit Ref"=w321:refnum<vi>, "Settings Ref"=w320:refnum<vi>, "Data Ref"=w316:refnum<vi>)
        n122 = property class="WFChart (strict)"(reference=w316, "History Data"=waveform(dbl)[][] []) -> ()  [unwired: 1 in, 2 out]
        n123 = Build Array(w322, w321, w320) -> (w325:refnum<vi>[])
        n124 = Build Array(w318, w319) -> (w324:refnum<vi>[])
        n125 = call-poly "Enqueue Message.vi"("error in (no error)"=w313, "Message"="Broadcast settings", "Message Queue"=w314) -> ("error out"=w308:errorcluster, "dup Message Queue"=w309:refnum<queue>)  [unwired: 7 in]
        n126 = call "Set Enable State on Multiple Controls.vi"("Enable?"=TRUE, "Controls"=w324) -> ()  [unwired: 10 in]
        n127 = call "Set Enable State on Multiple Controls.vi"("Enable?"=FALSE, "Controls"=w325) -> ()  [unwired: 10 in]
        n128 = case shown="False" w310 {
          selector: w310 -> [_ w332]
          tunnel: [w331 w332] -> w307
          tunnel: w308 -> [w330 w333]
          tunnel: w309 -> [w328 _]
          tunnel: [w327 w333] -> w306
          frame False {
            w331 = TRUE  # Sequence Started?
            n129 = call-poly "Enqueue Message.vi"("error in (no error)"=w330, "Message"="Start Loops", "Message Queue"=w328) -> ("error out"=w327:errorcluster)  [unwired: 7 in, 1 out]
          }
          frame True {
          }
        }
        n130 = Merge Errors(w306) -> (w302:errorcluster)
        n131 = Unbundle By Name(w301) -> ("Feed Module Config.Process Name"=w305:string)
        n132 = Concatenate Strings(w305, " Sequence Start" ("text")) -> (w303:string)
        n133 = call "Write to Log File.vi"("error in"=w302, "text"=w303) -> ()  [unwired: 9 in, 1 out]
      }
      frame "Error" {
        # "Stop if there is an error"
        # "Error - Check the error message data and respond accordingly. This message is sent by the \"Error Handler\" VIs at the end of each loop in this application."
        n134 = Variant To Data(error in=w349, type=errorcluster {"status"=FALSE, "code"=0, "source"=""} ("error out"), Variant=w348) -> (data=w346:errorcluster, error out=w342:errorcluster)
        n135 = call <vilib>:"General Error Handler.vi"("error in (no error)"=w346) -> ("message"=w335:string)  [unwired: 10 in, 4 out]
        n136 = call-poly "Enqueue Message.vi"("Priority Message? (F)"=TRUE, "Message"="Exit", "Message Queue"=w345) -> ("error out"=w341:errorcluster)  [unwired: 7 in, 1 out]
        n137 = Merge Errors(w341, w342) -> (w334:errorcluster)
        n138 = Unbundle By Name(w336) -> ("Feed Module Config.Process Name"=w339:string)
        n139 = Concatenate Strings(w339, " Error: " ("text"), w335) -> (w337:string)
        n140 = call "Write to Log File.vi"("error in"=w334, "text"=w337) -> ()  [unwired: 9 in, 1 out]
      }
      frame "Exit" {
        w360 = TRUE  # Delete Module?
        # "Don't check the error outs. The acquisition and logging queues may have already been released."
        # "Close references owned by the Main VI."
        # "Stop the VI"
        # "Exit - Fire the User Event to stop the Event Handling Loop.  Also send Exit messages to the Acquisition and Logging loops."
        n141 = Release Queue(queue=w370, error in (no error)=w374) -> (error out=w368:errorcluster)  [unwired: 1 in, 2 out]
        n142 = call "Fire User Event - Stop.vi"("User Event - Stop"=w373) -> ("error out"=w372:errorcluster)  [unwired: 10 in]
        n143 = Release Notifier(notifier=w369, error in (no error)=w368) -> (error out=w367:errorcluster)  [unwired: 1 in, 2 out]
        n144 = Variant To Data(type=w360, Variant=w358) -> (data=w359:bool, error out=w361:errorcluster)  [unwired: 1 in]
        n145 = Build Array(w363) -> (w362:refnum<queue>[])
        n146 = Release Queue(queue=w365, error in (no error)=w367) -> (error out=w366:errorcluster)  [unwired: 1 in, 2 out]
        n147 = Select(t=w360, s=w361, f=w359) -> (s? t:f=w357:bool)
        n148 = for {
          tunnel: w362 -> [w381] mode=indexing
          # "Send the engine the stop, exit"
          n149 = call-poly "Enqueue Message.vi"("Message"="Stop", "Message Queue"=w381) -> ("dup Message Queue"=w382:refnum<queue>)  [unwired: 8 in, 1 out]
          n150 = call-poly "Enqueue Message.vi"("Message"="Exit", "Message Queue"=w382) -> ()  [unwired: 8 in, 2 out]
        }
        n151 = case "Don't enqueue Delete Module if opening campaign because it\nwill already have been deleted and new config loaded and we create\na race condition." shown="True" w357 {
          tunnel: w351 -> [_ w378]
          tunnel: w356 -> [_ w376]
          frame False {
          }
          frame True {
            n152 = Unbundle By Name(w378) -> ("Feed Module Config.GUID"=w377:string)
            n153 = call-poly "Enqueue Message.vi"("Message Data"=w377, "Message"="Delete Module", "Message Queue"=w376) -> ()  [unwired: 7 in, 2 out]
          }
        }
        n154 = Merge Errors(w372, w366) -> (w352:errorcluster)
        n155 = Unbundle By Name(w351) -> ("Feed Module Config.Process Name"=w355:string)
        n156 = Concatenate Strings(w355, " Exit" ("text")) -> (w353:string)
        n157 = call "Write to Log File.vi"("error in"=w352, "text"=w353) -> ()  [unwired: 9 in, 1 out]
      }
      frame "Init UI Refs" {
        # "Enable: Start, Exit, Settings\nDisable: Stop"
        # "Init UI Refs - Store control references for UI controls.  Also enable/disable controls appropriately."
        n158 = property class="VI"("Front Panel.Closeable"=TRUE ("Front Panel Window:Closeable")) -> ()  [unwired: 2 in, 2 out]
        n159 = control-ref of="Status"() -> (w388:refnum<vi>)
        n160 = control-ref of="Exit"() -> (w385:refnum<vi>)
        n161 = Bundle By Name(cluster=w391, "Status Ref"=w388, "Exit Ref"=w385) -> (w390:T20)
        n162 = Build Array(w385) -> (w387:refnum<vi>[])
        n163 = call "Set Enable State on Multiple Controls.vi"("Enable?"=TRUE, "Controls"=w387) -> ()  [unwired: 10 in]
      }
      frame "Initialize" {
        # "Initialize - Get configuration settings, then message the UI to initialize, and broadcast the settings to the other message loops."
        n164 = property class="VI" props=["FP.State"]() -> (reference out=w400:refnum<vi>)  [unwired: 2 in, 2 out]
        n165 = call-poly "Enqueue Message.vi"("error in (no error)"=w403, "Message"="Init UI Refs", "Message Queue"=w408) -> ("error out"=w406:errorcluster, "dup Message Queue"=w407:refnum<queue>)  [unwired: 7 in]
        n166 = call-poly "Enqueue Message.vi"("error in (no error)"=w406, "Message"="Broadcast Settings", "Message Queue"=w407) -> ("error out"=w414:errorcluster, "dup Message Queue"=w413:refnum<queue>)  [unwired: 7 in]
        n167 = call "Make Child and Move.vi"("Process Name"=w399, "Name of Parent Panel"=w402, "New Center Coords"=w401, "VI in"=w400) -> ()  [unwired: 8 in]
        n168 = call-poly "Enqueue Message.vi"("error in (no error)"=w414, "Message Data"="Ready..." ("Ready..."), "Message"="Update Status", "Message Queue"=w413) -> ("error out"=w395:errorcluster)  [unwired: 6 in, 1 out]
        n169 = Unbundle By Name(w394) -> ("Feed Module Config.Process Name"=w398:string)
        n170 = Concatenate Strings(w398, " Initialize" ("text")) -> (w396:string)
        n171 = call "Write to Log File.vi"("error in"=w395, "text"=w396) -> ()  [unwired: 9 in, 1 out]
      }
      frame "Sequence Update" {
        # "Update the Sequence settings from the Sequence Dialog"
        # "Launch the Settings Dialog when the user clicks the 'Settings' button."
        n172 = Unbundle By Name(w431) -> ("Feed Module Config"=w430:T4)
        n173 = Variant To Data(type=T24 {"Auto?"=TRUE, "Manual Entry"=0.0, "Setpoint"=0.0} ("Cluster"), Variant=w427) -> (data=w426:T24)  [unwired: 1 in, 1 out]
        n174 = Unbundle By Name(w426) -> ("Auto?"=w425:bool, "Manual Entry"=w424:dbl, "Setpoint"=w423:dbl)
        n175 = Bundle By Name(cluster=w430, "Settings.Auto?"=w425, "Settings.Manual Entry"=w424, "Settings.PID 2 Parameters.Setpoint"=w423) -> (w420:T4)
        n176 = Bundle By Name(cluster=w431, "Feed Module Config"=w420) -> (w415:T2)
        n177 = call-poly "Enqueue Message.vi"("Message"="Broadcast Settings", "Message Queue"=w429) -> ("error out"=w422:errorcluster)  [unwired: 8 in, 1 out]
        n178 = Merge Errors(w422) -> (w416:errorcluster)
        n179 = Unbundle By Name(w415) -> ("Feed Module Config.Process Name"=w419:string)
        n180 = Concatenate Strings(w419, " Sequence Update" ("text")) -> (w417:string)
        n181 = call "Write to Log File.vi"("error in"=w416, "text"=w417) -> ()  [unwired: 9 in, 1 out]
      }
      frame "Logging Stopped" {
        # "Logic for determining what action to take when the logging has stopped."
        n182 = case shown="\"Waiting for Exit (Acq Stopped)\"" w442 {
          selector: w442 -> [w445 _ _ _ _]
          tunnel: [w445 UI_State."Waiting for Exit (Log Stopped)" ("UI State") UI_State."Waiting for Stop (Log Stopped)" ("UI State") UI_State."Idle" ("UI State") UI_State."Idle" ("UI State")] -> w441
          tunnel: w440 -> [w444 w446 w448 w454 w460]
          tunnel: [w444 w446 w448 w453 w459] -> w435
          tunnel: w439 -> [_ _ _ w452 w458]
          frame Default {
          }
          frame "Waiting for Exit", "Waiting for Exit (Log Stopped)" {
          }
          frame "Waiting for Stop", "Waiting for Stop (Log Stopped)" {
          }
          frame "Waiting for Exit (Acq Stopped)" {
            # "If we are waiting to exit, and the acquisition has already stopped, then the \"Logging Stopped\" message indicates that it is time to exit."
            n183 = call-poly "Enqueue Message.vi"("Priority Message? (F)"=TRUE, "error in (no error)"=w454, "Message"="Exit", "Message Queue"=w452) -> ("error out"=w453:errorcluster)  [unwired: 6 in, 1 out]
          }
          frame "Waiting for Stop (Acq Stopped)" {
            # "If we are waiting to stop, and the acquisition has already stopped, then the \"Logging Stopped\" message indicates that it is time to stop."
            n184 = call-poly "Enqueue Message.vi"("error in (no error)"=w460, "Message Data"="Ready..." ("Message"), "Message"="Update Status", "Message Queue"=w458) -> ("error out"=w459:errorcluster)  [unwired: 6 in, 1 out]
          }
        }
        n185 = Unbundle By Name(w434) -> ("Feed Module Config.Process Name"=w438:string)
        n186 = Concatenate Strings(w438, " Logging Stopped" ("text")) -> (w436:string)
        n187 = call "Write to Log File.vi"("error in"=w435, "text"=w436) -> ()  [unwired: 9 in, 1 out]
      }
      frame "Open Operational Window" {
        # "Keep track of how many times \nthe window has been opened"
        # "Duplicate this frame when creating new messages.  Change this comment in the duplicated frame to describe this message."
        n188 = Unbundle By Name(w471) -> ("Feed Module Config"=w472:T4)
        n189 = Unbundle By Name(w472) -> ("OP Load Count"=w473:i32)
        n190 = Increment(x=w473) -> (x+1=w474:i32)
        n191 = Bundle By Name(cluster=w472, "OP Load Count"=w474) -> (w470:T4)
        n192 = Bundle By Name(cluster=w471, "Feed Module Config"=w470) -> (w469:T2)
        n193 = call-by-ref "?"("Main UI Message Queue"=w477, "UI State"=w468, "error in (no error)"=w467, "Graph Notifier"=w476, "Message Queues"=w475, "Feed Module State Cluster in"=w469) -> ("error out"=w463:errorcluster, "Feed Module State Cluster out"=w462:T2)  [unwired: 5 in, 3 out]
        n194 = Unbundle By Name(w462) -> ("Feed Module Config.Process Name"=w466:string)
        n195 = Concatenate Strings(w466, " Open OP Window" ("text")) -> (w464:string)
        n196 = call "Write to Log File.vi"("error in"=w463, "text"=w464) -> ()  [unwired: 9 in, 1 out]
      }
      frame "Start" {
        # "We only have one loop but i've kept this in anyway"
        # "Clear chart"
        # "Message Acquisition and Logging loops to start"
        # "Enable: Stop\nDisable: Start, Exit, Settings"
        # "Start - Enable/Disable buttons appropriately for an acquisition that has started, and update status display."
        n197 = Unbundle By Name(w503) -> ("Trigger Ref"=w494:refnum<vi>, "Stop Ref"=w495:refnum<vi>, "Start Ref"=w498:refnum<vi>, "Exit Ref"=w497:refnum<vi>, "Settings Ref"=w496:refnum<vi>, "Data Ref"=w485:refnum<vi>)
        n198 = property class="WFChart (strict)"(reference=w485, "History Data"=waveform(dbl)[][] []) -> ()  [unwired: 1 in, 2 out]
        n199 = Build Array(w498, w497, w496) -> (w501:refnum<vi>[])
        n200 = Build Array(w494, w495) -> (w500:refnum<vi>[])
        n201 = call-poly "Enqueue Message.vi"("error in (no error)"=w486, "Message"="Broadcast settings", "Message Queue"=w488) -> ("error out"=w489:errorcluster, "dup Message Queue"=w487:refnum<queue>)  [unwired: 7 in]
        n202 = call "Set Enable State on Multiple Controls.vi"("Enable?"=TRUE, "Controls"=w500) -> ()  [unwired: 10 in]
        n203 = call "Set Enable State on Multiple Controls.vi"("Enable?"=FALSE, "Controls"=w501) -> ()  [unwired: 10 in]
        n204 = call-poly "Enqueue Message.vi"("error in (no error)"=w489, "Message"="Start Loops", "Message Queue"=w487) -> ("error out"=w490:errorcluster)  [unwired: 7 in, 1 out]
        n205 = Merge Errors(w490) -> (w480:errorcluster)
        n206 = Unbundle By Name(w479) -> ("Feed Module Config.Process Name"=w483:string)
        n207 = Concatenate Strings(w483, " Start" ("text")) -> (w481:string)
        n208 = call "Write to Log File.vi"("error in"=w480, "text"=w481) -> ()  [unwired: 9 in, 1 out]
      }
      frame "Start Loops" {
        # "I'm not entirly sure where we would have a second Process Name in a module but i'm leaving it for now"
        # "Message Acquisition and Logging loops to start"
        # "Start - Enable/Disable buttons appropriately for an acquisition that has started, and update status display."
        n209 = Unbundle By Name(w504) -> ("Feed Module Config.Process Name"=w506:string)
        n210 = Build Array(w510) -> (w508:refnum<queue>[])
        n211 = for {
          tunnel: w507 -> [w516]
          tunnel: [w515] -> w509 mode=indexing
          tunnel: w508 -> [w514] mode=indexing
          tunnel: w506 -> [w513]
          n212 = call-poly "Enqueue Message.vi"("error in (no error)"=w516, "Message Data"=w513, "Message"="Start", "Message Queue"=w514) -> ("error out"=w515:errorcluster)  [unwired: 6 in, 1 out]
        }
        n213 = property class="VI"("Front Panel.Title"=w506) -> ()  [unwired: 2 in, 2 out]
        n214 = Merge Errors(w509) -> (w505:errorcluster)
      }
      frame "Start Log" {
        # "I'm not entirly sure where we would have a second Process Name in a module but i'm leaving it for now"
        # "Message Acquisition and Logging loops to start"
        # "Start - Enable/Disable buttons appropriately for an acquisition that has started, and update status display."
        n215 = Unbundle By Name(w518) -> ("Feed Module Config.Process Name"=w523:string)
        n216 = Build Array(w527) -> (w525:refnum<queue>[])
        n217 = for {
          tunnel: w524 -> [w533]
          tunnel: [w532] -> w526 mode=indexing
          tunnel: w525 -> [w531] mode=indexing
          tunnel: w523 -> [w530]
          n218 = call-poly "Enqueue Message.vi"("error in (no error)"=w533, "Message Data"=w530, "Message"="Start Log", "Message Queue"=w531) -> ("error out"=w532:errorcluster)  [unwired: 6 in, 1 out]
        }
        n219 = property class="VI"("Front Panel.Title"=w523) -> ()  [unwired: 2 in, 2 out]
        n220 = Merge Errors(w526) -> (w519:errorcluster)
        n221 = Unbundle By Name(w518) -> ("Feed Module Config.Process Name"=w522:string)
        n222 = Concatenate Strings(w522, " Start Log" ("text")) -> (w520:string)
        n223 = call "Write to Log File.vi"("error in"=w519, "text"=w520) -> ()  [unwired: 9 in, 1 out]
      }
      frame "Stop" {
        # "Stop Pauses the engine"
        # "Enable: Start, Exit, Settings\nDisable: Stop"
        # "Stop - Enable/Disable buttons appropriately for an acquisition that has stopped, and update status display."
        n224 = Unbundle By Name(w556) -> ("Trigger Ref"=w547:refnum<vi>, "Stop Ref"=w548:refnum<vi>, "Start Ref"=w551:refnum<vi>, "Exit Ref"=w550:refnum<vi>, "Settings Ref"=w549:refnum<vi>)
        n225 = call-poly "Enqueue Message.vi"("error in (no error)"=w544, "Message Data"="Ready..." ("Ready..."), "Message"="Update Status", "Message Queue"=w559) -> ("error out"=w542:errorcluster)  [unwired: 6 in, 1 out]
        n226 = Build Array(w551, w550, w549) -> (w554:refnum<vi>[])
        n227 = Build Array(w547, w548) -> (w553:refnum<vi>[])
        n228 = call-poly "Enqueue Message.vi"("error in (no error)"=w542, "Message"="Pause", "Message Queue"=w543) -> ("error out"=w540:errorcluster)  [unwired: 7 in, 1 out]
        n229 = call "Set Enable State on Multiple Controls.vi"("Enable?"=FALSE, "Controls"=w553) -> ()  [unwired: 10 in]
        n230 = call "Set Enable State on Multiple Controls.vi"("Enable?"=TRUE, "Controls"=w554) -> ()  [unwired: 10 in]
        n231 = case shown="\"Waiting for Exit\"" w545 {
          selector: w545 -> [_ w561]
          tunnel: [UI_State."Waiting for Stop" ("UI State") w561] -> w546
          frame Default {
          }
          frame "Waiting for Exit" {
          }
        }
        n232 = Merge Errors(w540) -> (w536:errorcluster)
        n233 = Unbundle By Name(w535) -> ("Feed Module Config.Process Name"=w539:string)
        n234 = Concatenate Strings(w539, "Stop" ("text")) -> (w537:string)
        n235 = call "Write to Log File.vi"("error in"=w536, "text"=w537) -> ()  [unwired: 9 in, 1 out]
      }
      frame "Update Status" {
        # "Update Display - Convert the message data to a string to display in the Status indicator."
        n236 = Unbundle By Name(w572) -> ("Trigger Ref"=w568:refnum<vi>, "Stop Ref"=w571:refnum<vi>)
        n237 = Variant To Data(error in=w576, type="", Variant=w575) -> (data=w569:string, error out=w573:errorcluster)
        "Status" <- w569
        n238 = property class="Bool"(reference=w571) -> ("DisabledEnum"=w570:T25)  [unwired: 1 in, 2 out]
        n239 = case shown="\"Enabled\"" w570 {
          tunnel: w569 -> [w579 _]
          tunnel: w568 -> [w580 _]
          frame "Enabled" {
            # "Disable the Force Trigger only while we are logging."
            n240 = Build Array(w580) -> (w581:refnum<vi>[])
            n241 = Not Equal?(x="Logging" ("Logging"), y=w579) -> (x != y?=w577:bool)
            n242 = call "Set Enable State on Multiple Controls.vi"("Enable?"=w577, "Controls"=w581) -> ()  [unwired: 10 in]
          }
          frame "Disabled", Default {
          }
        }
        n243 = Merge Errors(w573) -> (w563:errorcluster)
        n244 = Unbundle By Name(w562) -> ("Feed Module Config.Process Name"=w566:string)
        n245 = Concatenate Strings(w566, "Update Status" ("text")) -> (w564:string)
        n246 = call "Write to Log File.vi"("error in"=w563, "text"=w564) -> ()  [unwired: 9 in, 1 out]
      }
      frame Default {
        # "'Default' case only runs if there is a message that isn't defined in any of the other cases.  Output a programming error."
        n247 = xnode "Error Ring"("parameter 0"=w582) -> ("error out"=w584:errorcluster)
        n248 = Unbundle By Name(w583) -> ("Feed Module Config.Process Name"=w587:string)
        n249 = Concatenate Strings(w587, "Incorrect Message Recieved: " ("text"), w582) -> (w585:string)
        n250 = call "Write to Log File.vi"("error in"=w584, "text"=w585) -> ()  [unwired: 9 in, 1 out]
      }
    }
    n251 = call "Error Handler - Message Handling Loop.vi"("error in (no error)"=w146, "Message Queue"=w144) -> ("dup error in"=w145:errorcluster)  [unwired: 8 in, 1 out]
  }
  n252 = call "Main Loop.vi"("error in (no error)"=w5, "Chart Notifier"=w21, "Message Queues"=w22) -> ("error out"=w23:errorcluster)  [unwired: 8 in]
  n253 = Unregister For Events(event registration refnum=w31, error in=w37) -> (error out=w32:errorcluster)
  n254 = Close Reference(reference=w20) -> ()  [unwired: 1 in, 1 out]
  n255 = Merge Errors(w32, w38, w5, w23) -> (w36:errorcluster)
  n256 = call "Destroy User Event - Stop.vi"("error in (no error)"=w36, "User Event - Stop"=w34) -> ("error out"=w7:errorcluster)  [unwired: 9 in]
  n257 = flat-sequence {
    tunnel: w7 -> [_]
    frame #0 {
      n258 = invoke class="VI" method="FP.Close"() -> ()  [unwired: 3 in, 3 out]
    }
  }
